vi "CRYPick arrays to save.vi"(6 "Start of file":bool, 8 "axes":cluster{"x":bool, "y":bool, "z":bool}, 9 "Z":dbl[](array[numeric]) format="%.2f", 10 "Y":dbl[](array[numeric]) format="%.2f", 11 "X":dbl[](array[numeric]) format="%.2f") -> (3 "Data points to save":dbl[][](array[numeric]) format="%.2f")   [LabVIEW 2013]
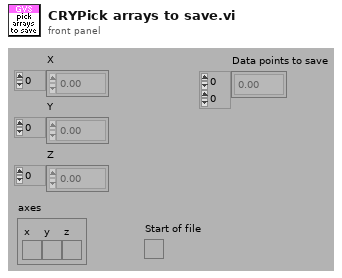
[diagram p1: front panel]
types:
  T1 = cluster{"Numeric":dbl, "Numeric":dbl, "Numeric":dbl}
  T2 = cluster{"Numeric":dbl, "Numeric":dbl, "Numeric":dbl}[]
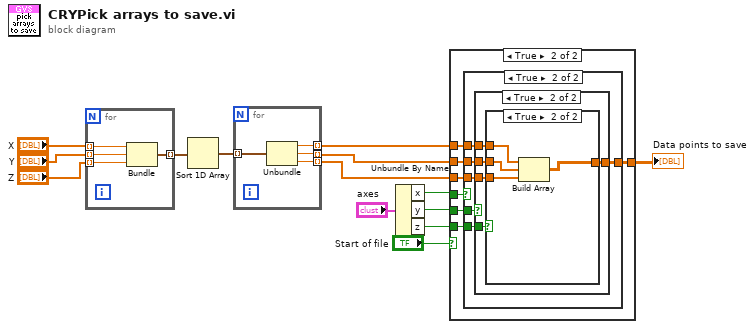
[diagram p0: block diagram]
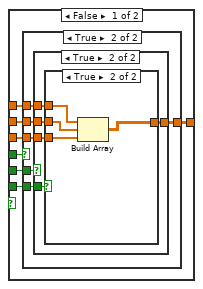
[diagram p2: hidden frame]
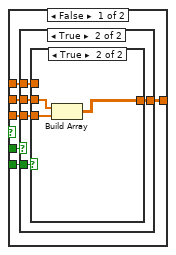
[diagram p3: hidden frame]
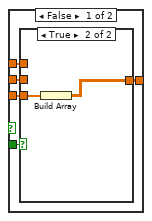
[diagram p4: hidden frame]
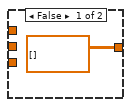
[diagram p5: hidden frame]
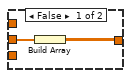
[diagram p6: hidden frame]
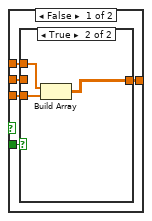
[diagram p7: hidden frame]
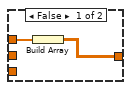
[diagram p8: hidden frame]
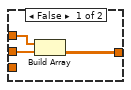
[diagram p9: hidden frame]
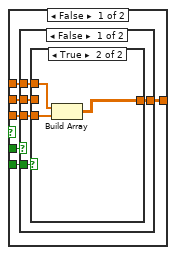
[diagram p10: hidden frame]
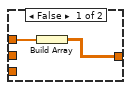
[diagram p11: hidden frame]
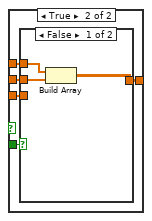
[diagram p12: hidden frame]
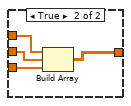
[diagram p13: hidden frame]
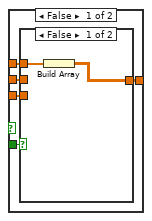
[diagram p14: hidden frame]
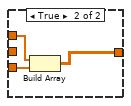
[diagram p15: hidden frame]
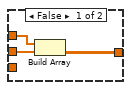
[diagram p16: hidden frame]
diagram:
  n1 = for {
    tunnel: "X" -> [w18] mode=indexing
    tunnel: "Y" -> [w17] mode=indexing
    tunnel: [w16] -> w8 mode=indexing
    tunnel: "Z" -> [w15] mode=indexing
    n2 = Bundle("Numeric"=w18, "Numeric"=w17, "Numeric"=w15) -> (w16:T1)  [unwired: 1 in]
  }
  n3 = Sort 1D Array(array=w8) -> (sorted array=w4:T2)
  n4 = for {
    tunnel: w4 -> [w22] mode=indexing
    tunnel: [w21] -> w3 mode=indexing
    tunnel: [w20] -> w2 mode=indexing
    tunnel: [w19] -> w1 mode=indexing
    n5 = Unbundle(w22) -> ("Numeric"=w21:dbl, "Numeric"=w20:dbl, "Numeric"=w19:dbl)
  }
  n6 = Unbundle By Name("axes") -> ("x"=w12:bool, "y"=w11:bool, "z"=w10:bool)
  n7 = case shown="True" "Start of file" {
    tunnel: w12 -> [w29 w88]
    tunnel: w11 -> [w28 w87]
    tunnel: w10 -> [w27 w86]
    tunnel: w3 -> [w26 w85]
    tunnel: w2 -> [w25 w84]
    tunnel: w1 -> [w24 w83]
    tunnel: [w23 w82] -> w9
    frame False {
      n8 = case shown="True" w29 {
        tunnel: w28 -> [w35 w59]
        tunnel: w27 -> [w34 w58]
        tunnel: w26 -> [w33 w57]
        tunnel: w25 -> [w32 w56]
        tunnel: w24 -> [w31 w55]
        tunnel: [w30 w54] -> w23
        frame False {
          n9 = case shown="True" w35 {
            tunnel: w34 -> [w40 w48]
            tunnel: w33 -> [w39 w47]
            tunnel: w32 -> [w38 w46]
            tunnel: w31 -> [w37 w45]
            tunnel: [w36 w44] -> w30
            frame False {
              n10 = case shown="True" w40 {
                tunnel: w39 -> [_ _]
                tunnel: w38 -> [_ _]
                tunnel: w37 -> [_ w43]
                tunnel: [dbl[][] [] w42] -> w36
                frame False {
                }
                frame True {
                  n11 = Build Array(w43) -> (w42:dbl[][])
                }
              }
            }
            frame True {
              n12 = case shown="True" w48 {
                tunnel: w47 -> [_ _]
                tunnel: w46 -> [w50 w51]
                tunnel: w45 -> [_ w53]
                tunnel: [w49 w52] -> w44
                frame False {
                  n13 = Build Array(w50) -> (w49:dbl[][])
                }
                frame True {
                  n14 = Build Array(w51, w53) -> (w52:dbl[][])
                }
              }
            }
          }
        }
        frame True {
          n15 = case shown="True" w59 {
            tunnel: w58 -> [w64 w74]
            tunnel: w57 -> [w63 w73]
            tunnel: w56 -> [w62 w72]
            tunnel: w55 -> [w61 w71]
            tunnel: [w60 w70] -> w54
            frame False {
              n16 = case shown="True" w64 {
                tunnel: w63 -> [w66 w67]
                tunnel: w62 -> [_ _]
                tunnel: w61 -> [_ w69]
                tunnel: [w65 w68] -> w60
                frame False {
                  n17 = Build Array(w66) -> (w65:dbl[][])
                }
                frame True {
                  n18 = Build Array(w67, w69) -> (w68:dbl[][])
                }
              }
            }
            frame True {
              n19 = case shown="True" w74 {
                tunnel: w73 -> [w75 w78]
                tunnel: w72 -> [w77 w79]
                tunnel: w71 -> [_ w81]
                tunnel: [w76 w80] -> w70
                frame False {
                  n20 = Build Array(w75, w77) -> (w76:dbl[][])
                }
                frame True {
                  n21 = Build Array(w78, w79, w81) -> (w80:dbl[][])
                }
              }
            }
          }
        }
      }
    }
    frame True {
      n22 = case shown="True" w88 {
        tunnel: w87 -> [w94 w122]
        tunnel: w86 -> [w93 w121]
        tunnel: w85 -> [w92 w120]
        tunnel: w84 -> [w91 w119]
        tunnel: w83 -> [w90 w118]
        tunnel: [w89 w117] -> w82
        frame False {
          n23 = case shown="False" w94 {
            tunnel: w93 -> [w99 w109]
            tunnel: w92 -> [w98 w108]
            tunnel: w91 -> [w97 w107]
            tunnel: w90 -> [w96 w106]
            tunnel: [w95 w105] -> w89
            frame False {
              n24 = case shown="True" w99 {
                tunnel: w98 -> [w101 w102]
                tunnel: w97 -> [_ _]
                tunnel: w96 -> [_ w104]
                tunnel: [w100 w103] -> w95
                frame False {
                  n25 = Build Array(w101) -> (w100:dbl[][])
                }
                frame True {
                  n26 = Build Array(w102, w104) -> (w103:dbl[][])
                }
              }
            }
            frame True {
              n27 = case shown="False" w109 {
                tunnel: w108 -> [w110 w113]
                tunnel: w107 -> [w112 w114]
                tunnel: w106 -> [_ w116]
                tunnel: [w111 w115] -> w105
                frame False {
                  n28 = Build Array(w110, w112) -> (w111:dbl[][])
                }
                frame True {
                  n29 = Build Array(w113, w114, w116) -> (w115:dbl[][])
                }
              }
            }
          }
        }
        frame True {
          n30 = case shown="True" w122 {
            tunnel: w121 -> [w127 w137]
            tunnel: w120 -> [w126 w136]
            tunnel: w119 -> [w125 w135]
            tunnel: w118 -> [w124 w134]
            tunnel: [w123 w133] -> w117
            frame False {
              n31 = case shown="False" w127 {
                tunnel: w126 -> [w129 w130]
                tunnel: w125 -> [_ _]
                tunnel: w124 -> [_ w132]
                tunnel: [w128 w131] -> w123
                frame False {
                  n32 = Build Array(w129) -> (w128:dbl[][])
                }
                frame True {
                  n33 = Build Array(w130, w132) -> (w131:dbl[][])
                }
              }
            }
            frame True {
              n34 = case shown="True" w137 {
                tunnel: w136 -> [w138 w141]
                tunnel: w135 -> [w140 w142]
                tunnel: w134 -> [_ w144]
                tunnel: [w139 w143] -> w133
                frame False {
                  n35 = Build Array(w138, w140) -> (w139:dbl[][])
                }
                frame True {
                  n36 = Build Array(w141, w142, w144) -> (w143:dbl[][])
                }
              }
            }
          }
        }
      }
    }
  }
  "Data points to save" <- w9
